vi "Channel Source Power Get Calibration Array.vi"(7 "RetValBufferSize":i32, 8 "error in (no error)":errorcluster {"code" format="%.0x"}, 9 "PortVal":i32 format="%.0g", 10 "RepCapIdentifier":string, 11 "instrument handle":refnum<k15>) -> (0 "error out":errorcluster {"code" format="%.0x"}, 1 "RetValActualSize":i32, 2 "RetVal":dbl[](array[numeric]) format="%.2p", 3 "instrument handle out":refnum<k15>)   [LabVIEW 2014, in "Agilent NA.lvlib"]
doc: "Gets the source power calibration array for the port."
uses:
  Agilent NA.lvlib
  AgNA.dll
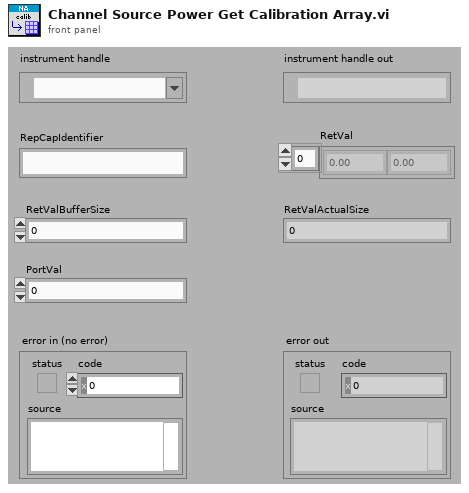
[diagram p1: front panel]
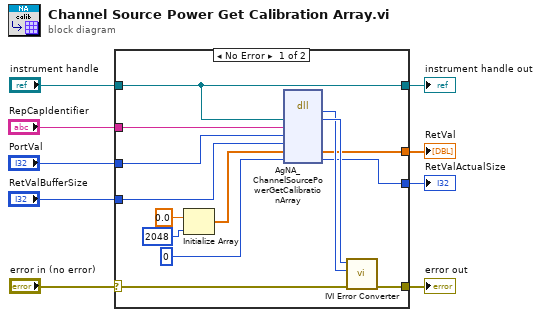
[diagram p0: block diagram]
diagram:
  n1 = case shown="No Error" "error in (no error)" {
    selector: "error in (no error)" -> [w21 w25]
    tunnel: [w20 w25] -> w9
    tunnel: "RepCapIdentifier" -> [w19 _]
    tunnel: "PortVal" -> [w18 _]
    tunnel: "RetValBufferSize" -> [w17 _]
    tunnel: [w13 _] -> w4
    tunnel: [w11 _] -> w3
    tunnel: "instrument handle" -> [w10 w24]
    tunnel: [w10 w24] -> w1
    frame No Error {
      n2 = Initialize Array(0.0 ("element"), 2048 ("dimension size")) -> (w16:dbl[])
      n3 = dll-call lib="AgNA**.dll" fn="AgNA_ChannelSourcePowerGetCalibrationArray"("Vi"=w10, "RepCapIdentifier"=w19, "PortVal"=w18, "RetValBufferSize"=w17, "RetVal"=w16, "RetValActualSize"=0) -> (w22:i32, "Vi"=w23:u32, "RetVal"=w13:dbl[], "RetValActualSize"=w11:i32)  [unwired: 6 in, 2 out]
      n4 = call "IVI Error Converter.vi"("error in (no error)"=w21, "IVI error code (0)"=w22, "instrument handle"=w23) -> ("error out"=w20:errorcluster)  [unwired: 7 in, 1 out]
    }
    frame Error {
    }
  }
  "error out" <- w9
  "instrument handle out" <- w1
  "RetVal" <- w4
  "RetValActualSize" <- w3
